vi "Add (Elementwise) - CM,C.vi"(1 "Complex Scalar c":cdb, 2 "Complex Matrix A":T1) -> (0 "A + c":T1)   [LabVIEW 2020, in "NI_Matrix.lvlib"]
doc: "Computes the sum of the inputs."
uses:
  <vilib>/Analysis/Matrix/NI_Matrix.lvlib
  <vilib>/Analysis/Matrix/Datatypes/ComplexMatrix.ctl
  <vilib>/Analysis/Matrix/Numeric/Conversions/Matrix To Array - CM.vi
  <vilib>/Analysis/Matrix/Numeric/Conversions/Array To Matrix - CA2.vi
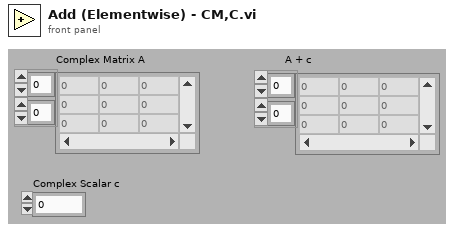
[diagram p1: front panel]
types:
  T1 = typedef "NI_Matrix.lvlib/ComplexMatrix.ctl" = cdb[][]
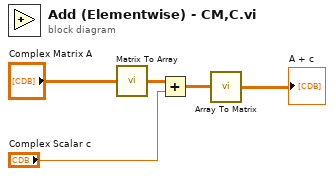
[diagram p0: block diagram]
diagram:
  n1 = call-poly <vilib>:"Matrix To Array.vi"("Complex Matrix"="Complex Matrix A") -> ("Complex 2D Array"=w4:cdb[][])
  n2 = Add(x=w4, y="Complex Scalar c") -> (x+y=w2:cdb[][])
  n3 = call-poly <vilib>:"Array To Matrix.vi"("Complex 2D Array"=w2) -> ("Complex Matrix"=→"A + c":T1)
